vi "Strip Qualified Name.vi"(2 "name":string) -> (5 "stripped name":string, 7 "last name":string)   [LabVIEW 2021, in "MeasurementService Editor.lvlib"]
uses:
  MeasurementService Editor.lvlib
  <vilib>/regexp/Match Regular Expression.xnode
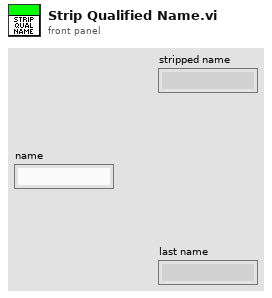
[diagram p1: front panel]
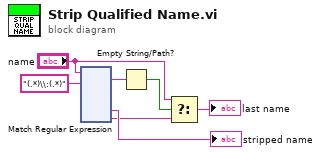
[diagram p0: block diagram]
diagram:
  n1 = xnode "Match Regular Expression"("input string"="name", "regular expression"="(.*)\\:(.*)") -> ("whole match"=w5:string, "submatch 1"=→"stripped name":string, "submatch 2"=w2:string)  [unwired: 4 in, 4 out]
  n2 = Empty String/Path?(string/path=w5) -> (empty?=w4:bool)
  n3 = Select(t="name", s=w4, f=w2) -> (s? t:f=→"last name":string)
